vi "SL2_AD_DLL_Phoibos_ListDeviceModes.vi"(0 "dll path in":path, 1 "dev_type":T1, 2 "pHandle":u32, 3 "error in":errorcluster) -> (5 "dll path out":path, 6 "modeIDs":u32[](array[numeric]), 7 "devicemodes":string[](array[string]), 8 "error out":errorcluster)   [LabVIEW 2020]
uses:
  DEFINITIONS/DEF_dev_type.ctl
  DEFINITIONS/DEF_T_error_enum.ctl
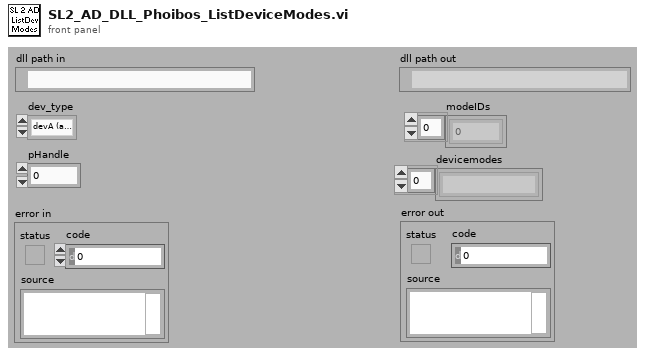
[diagram p1: front panel]
types:
  T1 = typedef "DEF_dev_type.ctl" = enum32{"devA (analyzer)", "devD (detector)"}
  T2 = typedef "DEF_T_error_enum.ctl" = u32
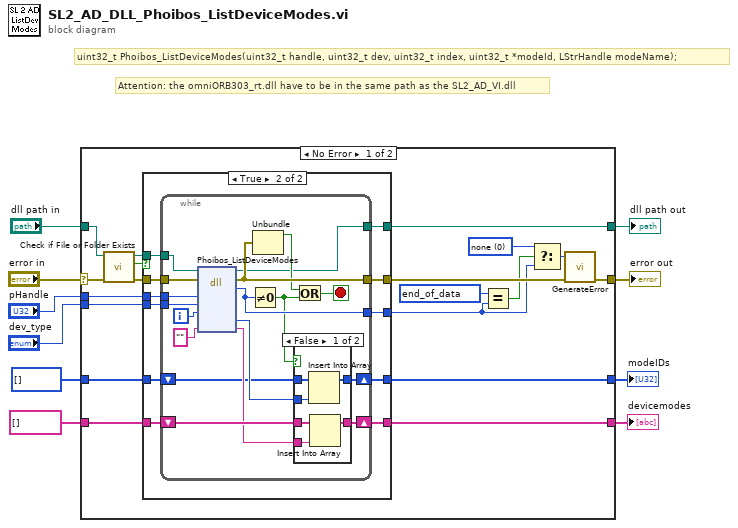
[diagram p0: block diagram]
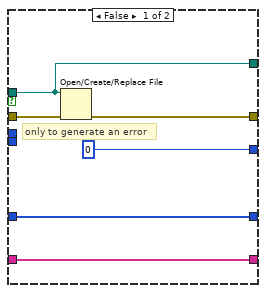
[diagram p2: hidden frame]
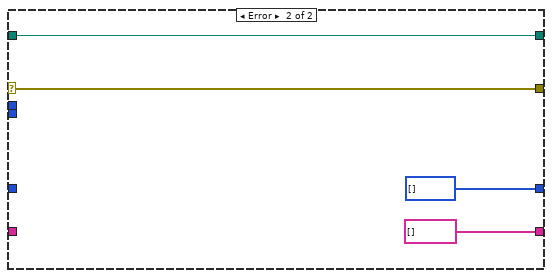
[diagram p4: hidden frame]
diagram:
  # "uint32_t Phoibos_ListDeviceModes(uint32_t handle, uint32_t dev, uint32_t index, uint32_t *modeId, LStrHandle modeName);"
  # "Attention: the omniORB303_rt.dll have to be in the same path as the SL2_AD_VI.dll"
  n1 = case shown="No Error" "error in" {
    selector: "error in" -> [w27 w75]
    tunnel: [w29 string[] [] ("Array")] -> w10
    tunnel: [w19 w75] -> w9
    tunnel: [w28 w76] -> w8
    tunnel: "dll path in" -> [w26 w76]
    tunnel: "dev_type" -> [w25 _]
    tunnel: "pHandle" -> [w24 _]
    tunnel: [w23 u32[] [] ("Array")] -> w3
    tunnel: u32[] [] ("Array") -> [w22 _]
    tunnel: string[] [] ("Array") -> [w21 _]
    frame No Error {
      w14 = T2 8388608 items=["none"=0, "busy"=65536, "error"=131072, "parameter"=262144, "locked"=524288, "sync"=1048576, "connection"=2097152, "internal"=4194304, "end_of_data"=8388608] ("DEF_T_error_enum")
      w17 = T2 0 items=["none"=0, "busy"=65536, "error"=131072, "parameter"=262144, "locked"=524288, "sync"=1048576, "connection"=2097152, "internal"=4194304, "end_of_data"=8388608] ("DEF_T_error_enum")
      n2 = call <vilib>:"Check if File or Folder Exists.vi"("error in (no error)"=w27, "path"=w26) -> ("error out"=w11:errorcluster, "file or folder exists?"=w13:bool, "dup path"=w12:path)  [unwired: 7 in]
      n3 = case shown="True" w13 {
        tunnel: [w34 w46] -> w29
        tunnel: [w32 w45] -> w20
        tunnel: [0 ("error_code") w44] -> w15
        tunnel: [w31 w43] -> w28
        tunnel: w12 -> [w31 w42]
        tunnel: w11 -> [w33 w41]
        tunnel: w21 -> [w34 w40]
        tunnel: w25 -> [_ w39]
        tunnel: w24 -> [_ w38]
        tunnel: [w30 w37] -> w23
        tunnel: w22 -> [w30 w36]
        frame False {
          # "only to generate an error"
          n4 = Open/Create/Replace File(file path (use dialog)=w31, error in=w33) -> (error out=w32:errorcluster)  [unwired: 4 in, 2 out]
        }
        frame True {
          n5 = while {
            tunnel: [w62] -> w44
            tunnel: [w55] -> w45
            shift-right: [w61] -> w46
            shift-left: w40 -> [w60]
            tunnel: w42 -> [w58]
            tunnel: w41 -> [w53]
            tunnel: [w52] -> w43
            tunnel: w39 -> [w51]
            tunnel: w38 -> [w50]
            shift-right: [w47] -> w37
            shift-left: w36 -> [w48]
            i -> [w63]
            stop <- w57 stop-if-true
            n6 = dll-call lib="C:/Programme/SPECS/SpecsLab2/programming/LabView7.1/SL2_AD_VI.dll" fn="Phoibos_ListDeviceModes"(path in=w58, error in=w53, "pHandle"=w50, "dev_type"=w51, "index"=w63, "modename"="") -> (path out=w52:path, error out=w55:errorcluster, "error_code"=w62:u32, "modeID"=w49:u32, "modename"=w59:string)  [unwired: 5 in]
            n7 = Not Equal To 0?(x=w62) -> (x != 0?=w56:bool)
            n8 = Unbundle(w55) -> ("status"=w54:bool)  [unwired: 2 out]
            n9 = case shown="False" w56 {
              tunnel: [w70 w72] -> w61
              tunnel: w60 -> [w68 w72]
              tunnel: w59 -> [w69 _]
              tunnel: w49 -> [w67 _]
              tunnel: w48 -> [w66 w71]
              tunnel: [w65 w71] -> w47
              frame False {
                n10 = Insert Into Array(array=w66, new element=w67) -> (w65:u32[])  [unwired: 1 in]
                n11 = Insert Into Array(array=w68, new element=w69) -> (w70:string[])  [unwired: 1 in]
              }
              frame True {
              }
            }
            n12 = Or(x=w54, y=w56) -> (x .or. y?=w57:bool)
          }
        }
      }
      n13 = Equal?(x=w14, y=w15) -> (x = y?=w16:bool)
      n14 = Select(t=w17, s=w16, f=w15) -> (s? t:f=w18:T2)
      n15 = call "GenerateError.vi"("error in"=w20, "error_code"=w18) -> ("error out"=w19:errorcluster)  [unwired: 9 in]
    }
    frame Error {
    }
  }
  "devicemodes" <- w10
  "error out" <- w9
  "dll path out" <- w8
  "modeIDs" <- w3
